vi "ReadParent_header.vi"(8 "error in (no error)":errorcluster, 11 "object in":refnum<class "Message Class.lvclass">) -> (0 "error out":errorcluster, 2 "parent_header":T1={"msg_id"="", "username"="", "session"="", "date"=timestamp(0 s since 1904-01-01), "msg_type"="", "version"="5.0"}, 3 "object out":refnum<class "Message Class.lvclass">)   [LabVIEW 2018, in "ClientMessaging.lvlib" / "Message Class.lvclass"]
uses:
  Message Class.lvclass
  protected/header_dict.ctl
  Message Class.lvclass/Message Class.ctl
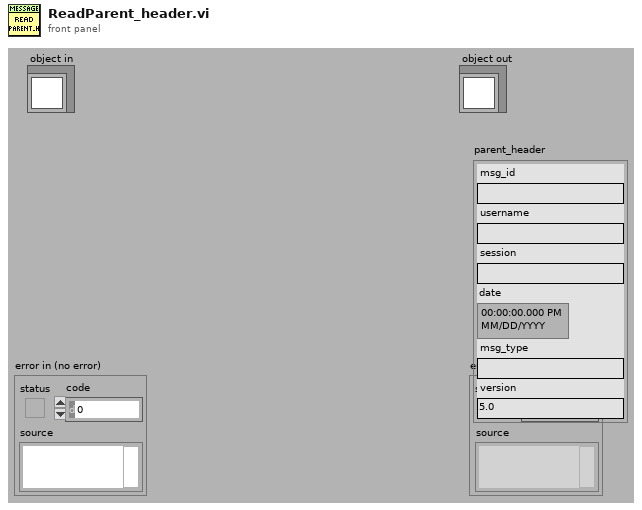
[diagram p1: front panel]
types:
  T1 = typedef "ClientMessaging.lvlib/Message Class.lvclass/header_dict.ctl" = cluster{"msg_id":string, "username":string, "session":string, "date":timestamp, "msg_type":string, "version":string}
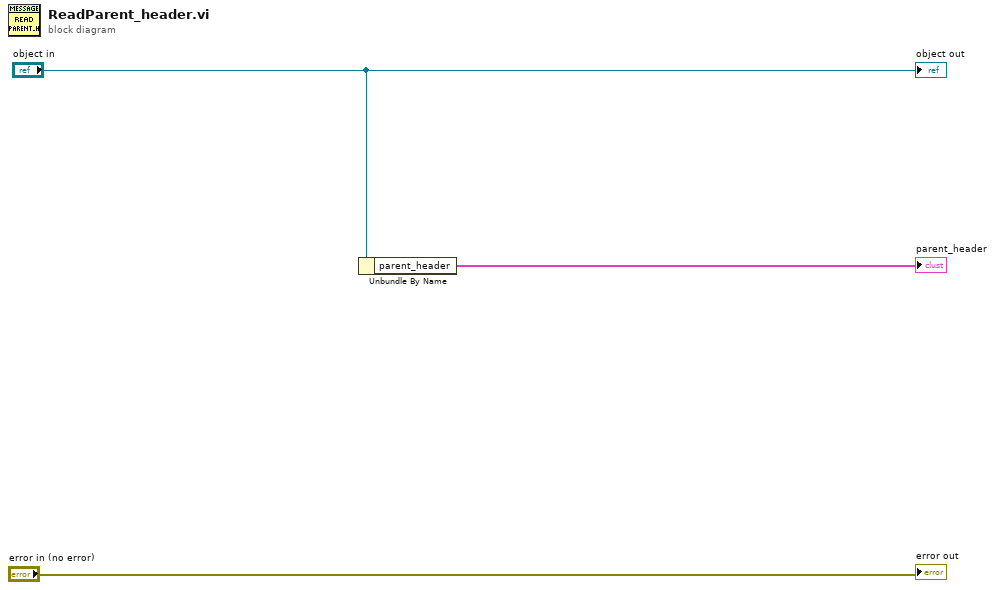
[diagram p0: block diagram]
diagram:
  n1 = Unbundle By Name("object in") -> ("parent_header"=→"parent_header":T1)
  "error out" <- "error in (no error)"
  "object out" <- "object in"
